vi "Launcher.vi"   [LabVIEW 2012, in "Win8uiFramework.lvlib"]
uses:
  Win8uiFramework.lvlib
  MainController.lvclass
  <vilib>/ActorFramework/Message Queue/Message Queue.lvclass/Message Queue.ctl
  <vilib>/ActorFramework/Actor/Actor.lvclass
  <vilib>/ActorFramework/Message Queue/Message Queue.lvclass
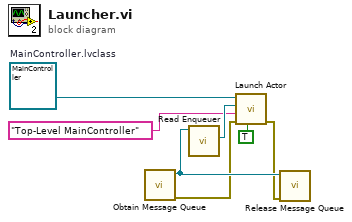
[diagram p0: block diagram]
diagram:
  w2 = refnum<class "MainController.lvclass"> refnum  # MainController.lvclass
  n1 = call <vilib>:"Obtain Message Queue.vi"() -> ("error out"=w4:errorcluster, "Message Queue"=w5:refnum<class "Message Queue.lvclass">)  [unwired: 10 in]
  n2 = call <vilib>:"Read Enqueuer.vi"("Message Queue"=w5) -> ("Message Enqueuer"=w7:refnum<class "Message Enqueuer.lvclass">)  [unwired: 10 in]
  n3 = call <vilib>:"Launch Actor.vi"("Open Actor Core front panel? (F)"=TRUE, "error in (no error)"=w4, "Actor Name"="Top-Level MainController", "Actor-to-Caller Enqueuer"=w7, "Actor"=w2) -> ("error out"=w3:errorcluster)  [unwired: 5 in, 1 out]
  n4 = call <vilib>:"Release Message Queue.vi"("error in (no error)"=w3, "Message Queue"=w5) -> ()  [unwired: 8 in, 2 out]
